vi "get power.vi"(8 "error in (no error)":errorcluster, 11 "Power Meter in":refnum<class "Power Meter.lvclass">) -> (0 "error out":errorcluster, 2 "Power":dbl=-1.0, 3 "Power Meter out":refnum<class "Power Meter.lvclass">)   [LabVIEW 2023, in "Power Meter.lvlib" / "Power Meter.lvclass"]
uses:
  Power Meter.lvclass
  C:/Program Files/National Instruments/LabVIEW 2023/vi.lib/ActorFramework/Actor/Actor.lvclass
  Power Meter.lvclass/Power Meter.ctl
  <vilib>/ActorFramework/Actor/Actor.lvclass/Actor.ctl
  Application Messages/Read Laser Power Msg/Read Laser Power Msg.lvclass/Read Laser Power Msg.ctl
  <vilib>/ActorFramework/Message Enqueuer/Message Enqueuer.lvclass/Message Enqueuer.ctl
  <vilib>/ActorFramework/Message Enqueuer/Enqueue.vi
  Application Messages/Read Laser Power Msg/Read Laser Power Msg.lvclass
  C:/Program Files/National Instruments/LabVIEW 2023/vi.lib/ActorFramework/Message/Message.lvclass
  Resources/GLOBAL/GLOBAL Time-critical.vi
  <vilib>/ActorFramework/Message Priority Queue/Priority Enqueue.vi
  <vilib>/ActorFramework/Actor/Actor.lvclass
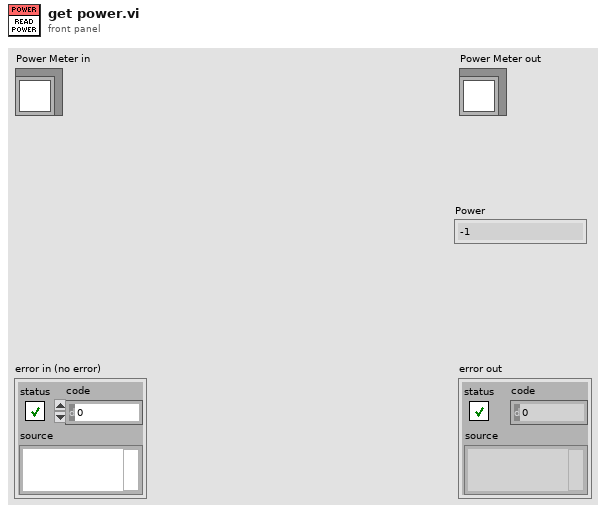
[diagram p1: front panel]
types:
  T1 = enum16{"Disabled", "Thorlabs", "Newport", "Coherent"}
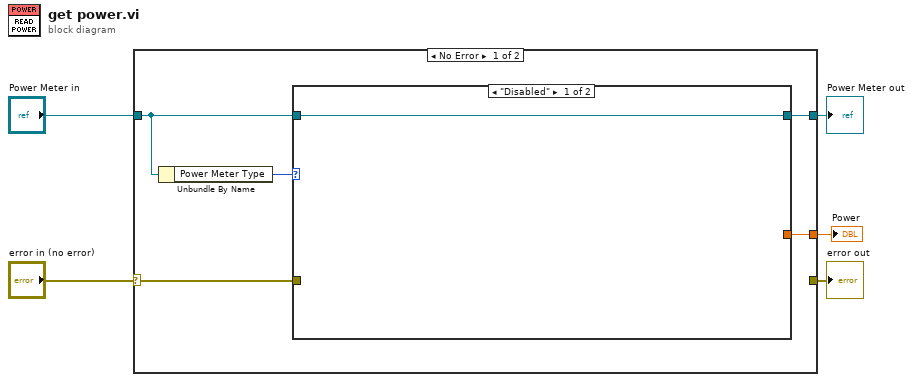
[diagram p0: block diagram]
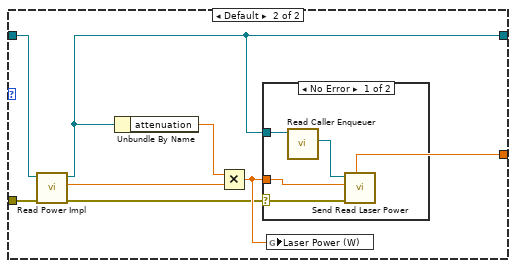
[diagram p2: hidden frame]
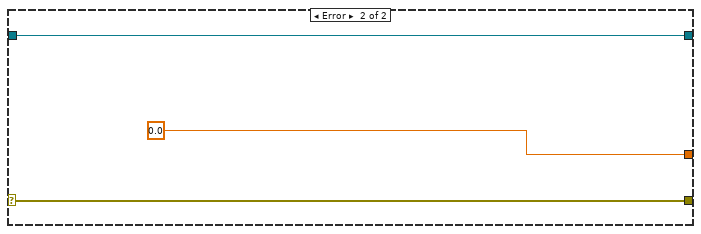
[diagram p4: hidden frame]
diagram:
  n1 = case shown="No Error" "error in (no error)" {
    selector: "error in (no error)" -> [w9 w25]
    tunnel: [_ w25] -> w4
    tunnel: [w8 w24] -> w2
    tunnel: "Power Meter in" -> [w7 w24]
    tunnel: [w10 0.0 ("Power")] -> w1
    frame No Error {
      n2 = Unbundle By Name(w7) -> ("Power Meter Type"=w6:T1)
      n3 = case shown="\"Disabled\"" w6 {
        tunnel: [_ w17] -> w10
        tunnel: w9 -> [_ w16]
        tunnel: w7 -> [w11 w14]
        tunnel: [w11 w13] -> w8
        frame "Disabled" {
        }
        frame Default {
          n4 = call-dynamic "Read Power Impl.vi"("error in (no error)"=w16, "Power Meter in"=w14) -> ("error out"=w15:errorcluster, "Raw Device Reading (W)"=w12:dbl, "Power Meter out"=w13:refnum<class "Power Meter.lvclass">)  [unwired: 7 in]
          n5 = Unbundle By Name(w13) -> ("attenuation"=w18:dbl)
          n6 = Multiply(x=w18, y=w12) -> (x*y=w17:dbl)
          n7 = case shown="No Error" w15 {
            selector: w15 -> [w20 _]
            tunnel: w17 -> [w21 _]
            tunnel: w13 -> [w19 _]
            frame No Error {
              n8 = call <vilib>:"Read Caller Enqueuer.vi"("Actor"=w19) -> ("Caller Enqueuer"=w22:refnum<class "Message Enqueuer.lvclass">)  [unwired: 10 in]
              n9 = call "Send Read Laser Power.vi"("error in (no error)"=w20, "Power"=w21, "Message Enqueuer"=w22) -> ()  [unwired: 7 in, 2 out]
            }
            frame Error {
              # "Ignore timeout errors"
            }
          }
          n10 = global write "GLOBAL Time-critical.vi" "Laser Power (W)"(w17) -> ()
        }
      }
    }
    frame Error {
    }
  }
  "error out" <- w4
  "Power Meter out" <- w2
  "Power" <- w1
